vi "DAQmx Reference Trigger (Analog Edge).vi"(0 "task/channels in":refnum<k21>, 5 "source":string, 7 "slope":i32(ring)=10280 items=["Rising"=10280, "Falling"=10171], 9 "level":dbl format="%0.2f", 11 "error in":errorcluster, 12 "pretrigger samples per channel":u32=500) -> (4 "task out":refnum<k21>, 15 "error out":errorcluster)   [LabVIEW 2011]
doc: "Configures the task to stop the acquisition when the device acquires all pretrigger samples; an analog signal reaches the level you specify; and the device acquires all post-trigger samples. When you use a Reference Trigger, the default for the read RelativeTo property is <B>First Pretrigger Sample</B> with a read Offset of 0."
uses:
  C:/Program Files/National Instruments/LabVIEW 2011/resource/objmgr/daqmx.rc
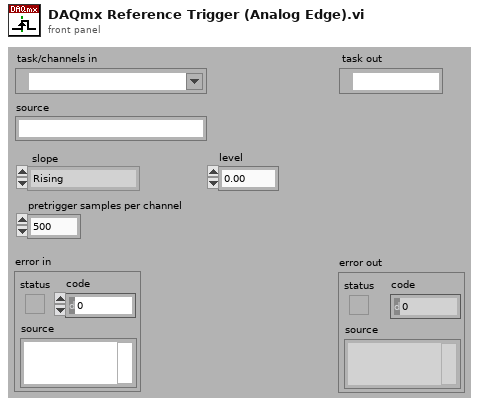
[diagram p1: front panel]
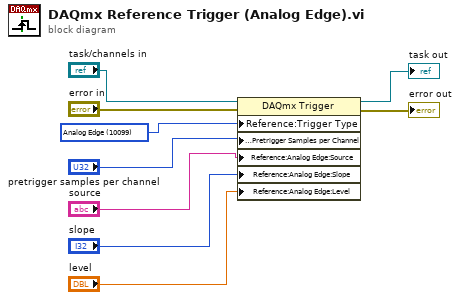
[diagram p0: block diagram]
diagram:
  w3 = 10099 items=["Analog Edge"=10099, "Digital Edge"=10150, "Analog Window"=10103, "None"=10230] ("Reference:Trigger Type")
  n1 = property class="DAQmx Trigger"(reference="task/channels in", error in="error in", "Reference:Trigger Type"=w3, "Reference:Pretrigger Samples per Channel"="pretrigger samples per channel", "Reference:Analog Edge:Source"="source", "Reference:Analog Edge:Slope"="slope", "Reference:Analog Edge:Level"="level") -> (reference out=→"task out":refnum<k21>, error out=→"error out":errorcluster)
